vi "Read Waveform.vi"(7 "Channel (0: CH 1)":u16(ring) items=["CH 1", "CH 2"], 8 "Error In (no error)":errorcluster, 9 "Number Of Points (1)":i16=1, 10 "Start Point (0)":i32, 11 "VISA Resource Name":refnum<visa-resource-name>) -> (0 "Error Out":errorcluster, 2 "Output Array":dbl[](array[numeric]) format="%.4e", 3 "VISA Resource Name Out":refnum<visa-resource-name>)   [LabVIEW 2010, in "Stanford Research 844.lvlib"]
doc: "This VI reads the points stored in the display buffers.\n\nNote: If data storage is set to Loop mode, be sure to pause data storage before reading any data. This is because the points are indexed relative to the oldest point, which is continually changing."
uses:
  <instrlib>/Stanford Research 844/Stanford Research 844.lvlib
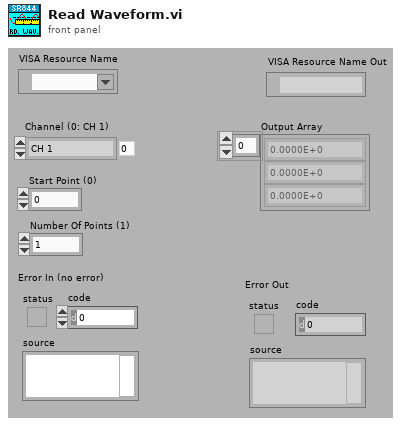
[diagram p1: front panel]
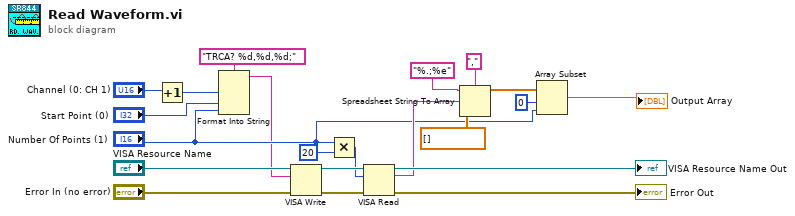
[diagram p0: block diagram]
diagram:
  n1 = Increment(x="Channel (0: CH 1)") -> (x+1=w17:u16)
  n2 = Format Into String(format string="TRCA? %d,%d,%d;", w17, "Start Point (0)", "Number Of Points (1)") -> (resulting string=w1:string)  [unwired: 2 in, 1 out]
  n3 = VISA Write(VISA resource name="VISA Resource Name", write buffer=w1, error in (no error)="Error In (no error)") -> (VISA resource name out=w16:refnum<visa-resource-name>, error out=w15:errorcluster)  [unwired: 1 out]
  n4 = Multiply(x="Number Of Points (1)", y=u32 20) -> (x*y=w10:u32)
  n5 = VISA Read(VISA resource name=w16, byte count=w10, error in (no error)=w15) -> (VISA resource name out=→"VISA Resource Name Out":refnum<visa-resource-name>, read buffer=w8:string, error out=→"Error Out":errorcluster)  [unwired: 1 out]
  n6 = Spreadsheet String To Array(delimiter (Tab)=",", format string="%.;%e", spreadsheet string=w8, array type (2D Dbl)=dbl[] []) -> (array=w5:dbl[])
  n7 = Array Subset(array=w5, index=0, length="Number Of Points (1)") -> (→"Output Array":dbl[])
